vi "Func-엑셀 데이터를 그래프로 출력.vi"() -> ()   [LabVIEW 2015] (continued)
65\t64.9\t75.27\n65\t64.91\t75.268\n65\t64.92\t75.265\n65\t64.93\t75.262\n65\t64.94\t75.262\n65\t64.95\t75.256\n65\t64.96\t75.249\n65\t64.97\t75.245\n65\t64.98\t75.237\n65\t65\t75.229\n65\t64.96\t75.224\n65\t64.96\t75.22\n65\t64.96\t75.216\n65\t64.96\t75.208\n65\t64.96\t75.205\n65\t64.96\t75.201\n65\t64.96\t75.197\n65\t64.96\t75.188\n65\t64.96\t75.185\n65\t64.96\t75.182\n65\t64.96\t75.17\n65\t64.97\t75.163\n65\t64.97\t75.157\n65\t64.97\t75.149\n65\t64.97\t75.143\n65\t64.97\t75.135\n65\t64.97\t75.135\n65\t64.97\t75.134\n65\t64.97\t75.125\n65\t64.97\t75.123\n65\t64.97\t75.118\n65\t64.97\t75.114\n65\t64.97\t75.107\n65\t64.97\t75.099\n65\t64.97\t75.093\n65\t64.97\t75.088\n65\t64.97\t75.082\n65\t64.97\t75.077\n65\t64.97\t75.071\n65\t64.97\t75.065\n65\t64.97\t75.059\n65\t64.97\t75.055\n65\t64.97\t75.052\n65\t64.97\t75.045\n65\t64.97\t75.038\n65\t64.97\t75.037\n65\t64.97\t75.034\n65\t64.97\t75.028\n65\t64.97\t75.023\n65\t64.97\t75.021\n65\t64.97\t75.017\n65\t64.98\t75.007\n65\t64.98\t75\n65\t64.98\t74.998\n65\t64.98\t74.991\n65\t64.98\t74.981\n65\t64.98\t74.977\n65\t64.98\t74.97\n65\t64.98\t74.965\n65\t64.98\t74.957\n65\t64.98\t74.952\n65\t64.98\t74.95\n65\t64.98\t74.948\n65\t64.98\t74.945\n65\t64.98\t74.943\n65\t64.98\t74.938\n65\t64.98\t74.928\n65\t64.98\t74.923\n65\t64.98\t74.909\n65\t64.98\t74.903\n65\t64.98\t74.896\n65\t64.98\t74.894\n65\t64.98\t74.891\n65\t64.98\t74.884\n65\t64.98\t74.88\n65\t64.98\t74.881\n65\t64.98\t74.88\n65\t64.98\t74.871\n65\t64.98\t74.869\n65\t64.98\t74.87\n65\t64.98\t74.864\n65\t64.98\t74.858\n65\t65\t74.853\n65\t65\t74.849\n65\t65\t74.846\n65\t65\t74.836\n65\t65\t74.829\n65\t65\t74.824\n65\t65\t74.812\n65\t65\t74.809\n65\t65\t74.802\n65\t65\t74.798\n65\t65\t74.795\n65\t65\t74.789\n65\t65\t74.786\n65\t65\t74.782\n65\t65\t74.778\n65\t65\t74.771\n65\t65\t74.766\n65\t65\t74.764\n65\t65\t74.755\n65\t65\t74.748\n65\t65\t74.743\n65\t65\t74.742\n65\t65\t74.74\n65\t65\t74.736\n65\t65\t74.735\n65\t65\t74.732\n65\t65\t74.725\n65\t65\t74.717\n65\t65\t74.713\n65\t65\t74.707\n65\t65\t74.7\n65\t65\t74.693\n65\t65\t74.689\n65\t65\t74.688\n65\t65\t74.684\n65\t65\t74.675\n65\t65\t74.672\n65\t65\t74.671\n65\t65\t74.666\n65\t65\t74.662\n65\t65\t74.657\n65\t65\t74.654\n65\t65\t74.652\n65\t65\t74.647\n65\t65\t74.638\n65\t65\t74.634\n65\t65\t74.628\n65\t65\t74.622\n65\t65\t74.616\n65\t65\t74.612\n65\t65\t74.602\n65\t65\t74.598\n65\t65\t74.596\n65\t65\t74.587\n65\t65\t74.581\n65\t65\t74.573\n65\t65\t74.572\n65\t65\t74.568\n65\t65\t74.561\n65\t65\t74.562\n65\t65\t74.56\n65\t65\t74.559\n65\t65\t74.559\n65\t65\t74.551\n65\t65\t74.547\n65\t65\t74.538\n65\t65\t74.537\n65\t65\t74.53\n65\t65\t74.523\n65\t65\t74.52\n65\t65\t74.513\n65\t65\t74.512\n65\t65\t74.506\n65\t65\t74.504\n65\t65\t74.5\n65\t65\t74.494\n65\t65\t74.489\n65\t65\t74.484\n65\t65\t74.477\n65\t65\t74.471\n65\t65\t74.467\n65\t65\t74.466\n65\t65\t74.462\n65\t65\t74.461\n65\t65\t74.454\n65\t65\t74.447\n65\t65\t74.444\n65\t65\t74.436\n65\t65\t74.431\n65\t65\t74.422\n65\t65\t74.42\n65\t65\t74.413\n65\t65\t74.41\n65\t65\t74.405\n65\t65\t74.403\n65\t65\t74.401\n65\t65\t74.395\n65\t65\t74.392\n65\t65\t74.386\n65\t65\t74.382\n65\t65\t74.377\n65\t65\t74.373\n65\t65\t74.368\n65\t65\t74.366\n65\t65\t74.362\n65\t65\t74.356\n65\t65\t74.355\n65\t65\t74.35\n65\t65\t74.347\n65\t65\t74.341\n65\t65\t74.336\n65\t65\t74.332\n65\t65\t74.328\n65\t65\t74.323\n65\t65\t74.323\n65\t65\t74.322\n65\t65\t74.315\n65\t65\t74.311\n65\t65\t74.301\n65\t65\t74.298\n65\t65\t74.292\n65\t65\t74.29\n65\t65\t74.289\n65\t65\t74.285\n65\t65\t74.279\n65\t65\t74.276\n65\t65\t74.27\n65\t65\t74.264\n65\t65\t74.257\n65\t65\t74.251\n65\t65\t74.247\n65\t65\t74.242\n65\t65\t74.238\n65\t65\t74.229\n65\t65\t74.23\n65\t65\t74.228\n65\t65\t74.229\n65\t65\t74.226\n65\t65\t74.222\n65\t65\t74.219\n65\t65\t74.212\n65\t65\t74.211\n65\t65\t74.201\n65\t65\t74.198\n65\t65\t74.196\n65\t65\t74.19\n65\t65\t74.186\n65\t65\t74.183\n65\t65\t74.179\n65\t65\t74.176\n65\t65\t74.17\n65\t65\t74.17\n65\t65\t74.165\n65\t65\t74.159\n65\t65\t74.155\n65\t65\t74.148\n65\t65\t74.139\n65\t65\t74.136\n65\t65\t74.134\n65\t65\t74.13\n65\t65\t74.127\n65\t65\t74.124\n65\t65\t74.123\n65\t65\t74.122\n65\t65\t74.116\n65\t65\t74.112\n65\t65\t74.108\n65\t65\t74.101\n65\t65\t74.099\n65\t65\t74.092\n65\t65\t74.088\n65\t65\t74.083\n65\t65\t74.078\n65\t65\t74.075\n65\t65\t74.074\n65\t65\t74.073\n65\t65\t74.068\n65\t65\t74.066\n65\t65\t74.061\n65\t65\t74.061\n65\t65\t74.053\n65\t65\t74.049\n65\t65\t74.049\n65\t65\t74.047\n65\t65\t74.045\n65\t65\t74.038\n65\t65\t74.037\n65\t65\t74.033\n65\t65\t74.025\n65\t65\t74.021\n65\t65\t74.016\n65\t65\t74.015\n65\t65\t74.011\n65\t65\t74.003\n65\t65\t74\n65\t65\t73.996\n65\t65\t73.987\n65\t65\t73.983\n65\t65\t73.982\n65\t65\t73.977\n65\t65\t73.975\n65\t65\t73.968\n65\t65\t73.963\n65\t65\t73.96\n65\t65\t73.956\n65\t65\t73.952\n65\t65\t73.949\n65\t65\t73.946\n65\t65\t73.946\n65\t65\t73.94\n65\t65\t73.933\n65\t65\t73.933\n65\t65\t73.928\n65\t65\t73.923\n65\t65\t73.923\n65\t65\t73.919\n65\t65\t73.916\n65\t65\t73.908\n65\t65\t73.904\n65\t65\t73.902\n65\t65\t73.895\n65\t65\t73.895\n65\t65\t73.892\n65\t65\t73.89\n65\t65\t73.889\n65\t65\t73.886\n65\t65\t73.884\n65\t65\t73.879\n65\t65\t73.873\n65\t65\t73.87\n65\t65\t73.864\n65\t65\t73.858\n65\t65\t73.855\n65\t65\t73.848\n65\t65\t73.845\n65\t65\t73.841\n65\t65\t73.839\n65\t65\t73.835\n65\t65\t73.833\n65\t65\t73.83\n65\t65\t73.831\n65\t65\t73.827\n65\t65\t73.823\n65\t65\t73.82\n65\t65\t73.809\n65\t65\t73.804\n65\t65\t73.798\n65\t65\t73.793\n65\t65\t73.787\n65\t65\t73.787\n65\t65\t73.788\n65\t65\t73.787\n65\t65\t73.784\n65\t65\t73.781\n65\t65\t73.78\n65\t65\t73.773\n65\t65\t73.766\n65\t65\t73.761\n65\t65\t73.757\n65\t65\t73.752\n65\t65\t73.747\n65\t65\t73.744\n65\t65\t73.743\n65\t65\t73.739\n65\t65\t73.736\n65\t65\t73.734\n65\t65\t73.73\n65\t65\t73.73\n65\t65\t73.729\n65\t65\t73.727\n65\t65\t73.724\n65\t65\t73.721\n65\t65\t73.716\n65\t65\t73.71\n65\t65\t73.705\n65\t65\t73.701\n65\t65\t73.697\n65\t65\t73.697\n65\t65\t73.697\n65\t65\t73.691\n65\t65\t73.686\n65\t65\t73.68\n65\t65\t73.675\n65\t65\t73.669\n65\t65\t73.664\n65\t65\t73.663\n65\t65\t73.662\n65\t65\t73.658\n65\t65\t73.654\n65\t65\t73.655\n65\t65\t73.649\n65\t65\t73.648\n65\t65\t73.644\n65\t65\t73.642\n65\t65\t73.641\n65\t65\t73.634\n65\t65\t73.632\n65\t65\t73.629\n65\t65\t73.625\n65\t65\t73.621\n65\t65\t73.614\n65\t65\t73.614\n65\t65\t73.61\n65\t65\t73.606\n65\t65\t73.605\n65\t65\t73.602\n65\t65\t73.6\n65\t65\t73.592\n65\t65\t73.585\n65\t65\t73.581\n65\t65\t73.572\n65\t65\t73.571\n65\t65\t73.572\n65\t65\t73.569\n65\t65\t73.572\n65\t65\t73.575\n65\t65\t73.576\n65\t65\t73.573\n65\t65\t73.572\n65\t65\t73.57\n65\t65\t73.562\n65\t65\t73.555\n65\t65\t73.549\n65\t65\t73.544\n65\t65\t73.539\n65\t65\t73.535\n65\t65\t73.537\n65\t65\t73.53\n65\t65\t73.528\n65\t65\t73.524\n65\t65\t73.518\n65\t65\t73.513\n65\t65\t73.51\n65\t65\t73.509\n65\t65\t73.506\n65\t65\t73.501\n65\t65\t73.497\n65\t65\t73.493\n65\t65\t73.486\n65\t65\t73.482\n65\t65\t73.477\n65\t65\t73.479\n65\t65\t73.474\n65\t65\t73.475\n65\t65\t73.474\n65\t65\t73.471\n65\t65\t73.471\n65\t65\t73.466\n65\t65\t73.46\n65\t65\t73.457\n65\t65\t73.45\n65\t65\t73.444\n65\t65\t73.442\n65\t65\t73.443\n65\t65\t73.446\n65\t65\t73.445\n65\t65\t73.443\n65\t65\t73.439\n65\t65\t73.434\n65\t65\t73.427\n65\t65\t73.421\n65\t65\t73.413\n65\t65\t73.407\n65\t65\t73.41\n65\t65\t73.405\n65\t65\t73.406\n65\t65\t73.406\n65\t65\t73.408\n65\t65\t73.407\n65\t65\t73.403\n65\t65\t73.402\n65\t65\t73.396\n65\t65\t73.393\n65\t65\t73.389\n65\t65\t73.386\n65\t65\t73.382\n65\t65\t73.377\n65\t65\t73.373\n65\t65\t73.37\n65\t65\t73.365\n65\t65\t73.364\n65\t65\t73.363\n65\t65\t73.361\n65\t65\t73.359\n65\t65\t73.356\n65\t65\t73.355\n65\t65\t73.354\n65\t65\t73.351\n65\t65\t73.345\n65\t65\t73.343\n65\t65\t73.338\n65\t65\t73.326\n65\t65\t73.32\n65\t65\t73.314\n65\t65\t73.315\n65\t65\t73.312\n65\t65\t73.313\n65\t65\t73.316\n65\t65\t73.31\n65\t65\t73.305\n65\t65\t73.299\n65\t65\t73.294\n65\t65\t73.286\n65\t65\t73.282\n65\t65\t73.284\n65\t65\t73.283\n65\t65\t73.282\n65\t65\t73.284\n65\t65\t73.28\n65\t65\t73.279\n65\t65\t73.277\n65\t65\t73.275\n65\t65\t73.273\n65\t65\t73.266\n65\t65\t73.265\n65\t65\t73.263\n65\t65\t73.257\n65\t65\t73.251\n65\t65\t73.246\n65\t65\t73.244\n65\t65\t73.242\n65\t65\t73.238\n65\t65\t73.236\n65\t65\t73.236\n65\t65\t73.233\n65\t65\t73.232\n65\t65\t73.227\n65\t65\t73.226\n65\t65\t73.219\n65\t65\t73.213\n65\t65\t73.209\n65\t65\t73.205\n65\t65\t73.204\n65\t65\t73.201\n65\t65\t73.201\n65\t65\t73.205\n65\t65\t73.2\n65\t65\t73.195\n65\t65\t73.194\n65\t65\t73.19\n65\t65\t73.187\n65\t65\t73.181\n65\t65\t73.182\n65\t65\t73.183\n65\t65\t73.18\n65\t65\t73.175\n65\t65\t73.173\n65\t65\t73.17\n65\t65\t73.168\n65\t65\t73.164\n65\t65\t73.165\n65\t65\t73.162\n65\t65\t73.158\n65\t65\t73.156\n65\t65\t73.155\n65\t65\t73.154\n65\t65\t73.15\n65\t65\t73.148\n65\t65\t73.148\n65\t65\t73.142\n65\t65\t73.139\n65\t65\t73.136\n65\t65\t73.127\n65\t65\t73.124\n65\t65\t73.122\n65\t65\t73.121\n65\t65\t73.113\n65\t65\t73.109\n65\t65\t73.109\n65\t65\t73.108\n65\t65\t73.101\n65\t65\t73.101\n65\t65\t73.1\n65\t65\t73.098\n65\t65\t73.101\n65\t65\t73.097\n65\t65\t73.098\n65\t65\t73.097\n65\t65\t73.098\n65\t65\t73.094\n65\t65\t73.089\n65\t65\t73.086\n65\t65\t73.078\n65\t65\t73.071\n65\t65\t73.068\n65\t65\t73.062\n65\t65\t73.056\n65\t65\t73.055\n65\t65\t73.052\n65\t65\t73.05\n65\t65\t73.047\n65\t65\t73.048\n65\t65\t73.048\n65\t65\t73.043\n65\t65\t73.037\n65\t65\t73.033\n65\t65\t73.028\n65\t65\t73.023\n65\t65\t73.02\n65\t65\t73.018\n65\t65\t73.02\n65\t65\t73.021\n65\t65\t73.017\n65\t65\t73.013\n65\t65\t73.015\n65\t65\t73.011\n65\t65\t73.009\n65\t65\t73\n65\t65\t72.997\n65\t65\t72.996\n65\t65\t72.988\n65\t65\t72.988\n65\t65\t72.986\n65\t65\t72.988\n65\t65\t72.988\n65\t65\t72.984\n65\t65\t72.983\n65\t65\t72.979\n65\t65\t72.977\n65\t65\t72.978\n65\t65\t72.976\n65\t65\t72.975\n65\t65\t72.972\n65\t65\t72.971\n65\t65\t72.968\n65\t65\t72.963\n65\t65\t72.96\n65\t65\t72.96\n65\t65\t72.957\n65\t65\t72.955\n65\t65\t72.949\n65\t65\t72.948\n65\t65\t72.945\n65\t65\t72.94\n65\t65\t72.936\n65\t65\t72.935\n65\t65\t72.935\n65\t65\t72.934\n65\t65\t72.932\n65\t65\t72.929\n65\t65\t72.932\n65\t65\t72.93\n65\t65\t72.928\n65\t65\t72.922\n65\t65\t72.917\n65\t65\t72.913\n65\t65\t72.909\n65\t65\t72.905\n65\t65\t72.902\n65\t65\t72.901\n65\t65\t72.901\n65\t65\t72.9\n65\t65\t72.893\n65\t65\t72.894\n65\t65\t72.891\n65\t65\t72.896\n65\t65\t72.893\n65\t65\t72.891\n65\t65\t72.891\n65\t65\t72.881\n65\t65\t72.881\n65\t65\t72.871\n65\t65\t72.871\n65\t65\t72.87\n65\t65\t72.87\n65\t65\t72.872\n65\t65\t72.868\n65\t65\t72.866\n65\t65\t72.863\n65\t65\t72.858\n65\t65\t72.854\n65\t65\t72.845\n65\t65\t72.845\n65\t65\t72.84\n65\t65\t72.838\n65\t65\t72.834\n65\t65\t72.833\n65\t65\t72.833\n65\t65\t72.829\n65\t65\t72.828\n65\t65\t72.822\n65\t65\t72.825\n65\t65\t72.824\n65\t65\t72.818\n65\t65\t72.816\n65\t65\t72.817\n65\t65\t72.819\n65\t65\t72.814\n65\t65\t72.809\n65\t65\t72.81\n65\t65\t72.811\n65\t65\t72.805\n65\t65\t72.796\n65\t65\t72.798\n65\t65\t72.796\n65\t65\t72.793\n65\t65\t72.786\n65\t65\t72.78\n65\t65\t72.777\n65\t65\t72.772\n65\t65\t72.772\n65\t65\t72.771\n65\t65\t72.773\n65\t65\t72.771\n65\t65\t72.776\n65\t65\t72.772\n65\t65\t72.768\n65\t65\t72.767\n65\t65\t72.761\n65\t65\t72.759\n65\t65\t72.755\n65\t65\t72.753\n65\t65\t72.751\n65\t65\t72.748\n65\t65\t72.751\n65\t65\t72.753\n65\t65\t72.751\n65\t65\t72.749\n65\t65\t72.745\n65\t65\t72.738\n65\t65\t72.733\n65\t65\t72.73\n65\t65\t72.724\n65\t65\t72.721\n65\t65\t72.721\n65\t65\t72.721\n65\t65\t72.719\n65\t65\t72.716\n65\t65\t72.72\n65\t65\t72.722\n65\t65\t72.72\n65\t65\t72.716\n65\t65\t72.717\n65\t65\t72.716\n65\t65\t72.709\n65\t65\t72.705\n65\t65\t72.705\n65\t65\t72.703\n65\t65\t72.697\n65\t65\t72.692\n65\t65\t72.691\n65\t65\t72.687\n65\t65\t72.682\n65\t65\t72.684\n65\t65\t72.689\n65\t65\t72.689\n65\t65\t72.682\n65\t65\t72.681\n65\t65\t72.68\n65\t65\t72.679\n65\t65\t72.673\n65\t65\t72.67\n65\t65\t72.671\n65\t65\t72.671\n65\t65\t72.667\n65\t65\t72.662\n65\t65\t72.657\n65\t65\t72.653\n65\t65\t72.652\n65\t65\t72.648\n65\t65\t72.647\n65\t65\t72.641\n65\t65\t72.644\n65\t65\t72.641\n65\t65\t72.64\n65\t65\t72.642\n65\t65\t72.639\n65\t65\t72.638\n65\t65\t72.636\n65\t65\t72.635\n65\t65\t72.632\n65\t65\t72.625\n65\t65\t72.62\n65\t65\t72.623\n65\t65\t72.62\n65\t65\t72.62\n65\t65\t72.619\n65\t65\t72.618\n65\t65\t72.616\n65\t65\t72.613\n65\t65\t72.61\n65\t65\t72.607\n65\t65\t72.605\n65\t65\t72.602\n65\t65\t72.601\n65\t65\t72.597\n65\t65\t72.595\n65\t65\t72.593\n65\t65\t72.59\n65\t65\t72.588\n65\t65\t72.585\n65\t65\t72.586\n65\t65\t72.584\n65\t65\t72.582\n65\t65\t72.581\n65\t65\t72.582\n65\t65\t72.581\n65\t65\t72.575\n65\t65\t72.572\n65\t65\t72.574\n65\t65\t72.57\n65\t65\t72.565\n65\t65\t72.566\n65\t65\t72.565\n65\t65\t72.562\n65\t65\t72.56\n65\t65\t72.555\n65\t65\t72.555\n65\t65\t72.551\n65\t65\t72.548\n65\t65\t72.549\n65\t65\t72.543\n65\t65\t72.544\n65\t65\t72.539\n65\t65\t72.54\n65\t65\t72.539\n65\t65\t72.536\n65\t65\t72.532\n65\t65\t72.529\n65\t65\t72.532\n65\t65\t72.526\n65\t65\t72.524\n65\t65\t72.522\n65\t65\t72.517\n65\t65\t72.519\n65\t65\t72.512\n65\t65\t72.514\n65\t65\t72.51\n65\t65\t72.51\n65\t65\t72.512\n65\t65\t72.506\n65\t65\t72.506\n65\t65\t72.501\n65\t65\t72.5\n65\t65\t72.493\n65\t65\t72.493\n65\t65\t72.493\n65\t65\t72.491\n65\t65\t72.493\n65\t65\t72.491\n65\t65\t72.492\n65\t65\t72.492\n65\t65\t72.488\n65\t65\t72.485\n65\t65\t72.478\n65\t65\t72.475\n65\t65\t72.47\n65\t65\t72.465\n65\t65\t72.467\n65\t65\t72.466\n65\t65\t72.467\n65\t65\t72.467\n65\t65\t72.466\n65\t65\t72.468\n65\t65\t72.464\n65\t65\t72.463\n65\t65\t72.463\n65\t65\t72.459\n65\t65\t72.452\n65\t65\t72.448\n65\t65\t72.445\n65\t65\t72.443\n65\t65\t72.44\n65\t65\t72.437\n65\t65\t72.439\n65\t65\t72.437\n65\t65\t72.434\n65\t65\t72.43\n65\t65\t72.428\n65\t65\t72.431\n65\t65\t72.434\n65\t65\t72.431\n65\t65\t72.429\n65\t65\t72.429\n65\t65\t72.424\n65\t65\t72.422\n65\t65\t72.421\n65\t65\t72.421\n65\t65\t72.42\n65\t65\t72.416\n65\t65\t72.418\n65\t65\t72.414\n65\t65\t72.408\n65\t65\t72.405\n65\t65\t72.406\n65\t65\t72.405\n65\t65\t72.399\n65\t65\t72.398\n65\t65\t72.4\n65\t65\t72.401\n65\t65\t72.397\n65\t65\t72.398\n65\t65\t72.402\n65\t65\t72.402\n65\t65\t72.396\n65\t65\t72.391\n65\t65\t72.391\n65\t65\t72.385\n65\t65\t72.379\n65\t65\t72.373\n65\t65\t72.37\n65\t65\t72.368\n65\t65\t72.367\n65\t65\t72.365\n65\t65\t72.366\n65\t65\t72.366\n65\t65\t72.367\n65\t65\t72.366\n65\t65\t72.364\n65\t65\t72.363\n65\t65\t72.36\n65\t65\t72.359\n65\t65\t72.358\n65\t65\t72.356\n65\t65\t72.355\n65\t65\t72.356\n65\t65\t72.358\n65\t65\t72.355\n65\t65\t72.352\n65\t65\t72.353\n65\t65\t72.345\n65\t65\t72.342\n65\t65\t72.336\n65\t65\t72.338\n65\t65\t72.337\n65\t65\t72.332\n65\t65\t72.331\n65\t65\t72.325\n65\t65\t72.324\n65\t65\t72.317\n65\t65\t72.316\n65\t65\t72.314\n65\t65\t72.318\n65\t65\t72.319\n65\t65\t72.317\n65\t65\t72.317\n65\t65\t72.312\n65\t65\t72.307\n65\t65\t72.303\n65\t65\t72.302\n65\t65\t72.299\n65\t65\t72.298\n65\t65\t72.295\n65\t65\t72.294\n65\t65\t72.296\n65\t65\t72.299\n65\t65\t72.3\n65\t65\t72.3\n65\t65\t72.298\n65\t65\t72.295\n65\t65\t72.293\n65\t65\t72.288\n65\t65\t72.281\n65\t65\t72.275\n65\t65\t72.28\n65\t65\t72.279\n65\t65\t72.276\n65\t65\t72.273\n65\t65\t72.271\n65\t65\t72.27\n65\t65\t72.268\n65\t65\t72.266\n65\t65\t72.264\n65\t65\t72.265\n65\t65\t72.271\n65\t65\t72.271\n65\t65\t72.266\n65\t65\t72.267\n65\t65\t72.267\n65\t65\t72.266\n65\t65\t72.257\n65\t65\t72.253\n65\t65\t72.254\n65\t65\t72.253\n65\t65\t72.248\n65\t65\t72.245\n65\t65\t72.245\n65\t65\t72.247\n65\t65\t72.243\n65\t65\t72.241\n65\t65\t72.239\n65\t65\t72.239\n65\t65\t72.24\n65\t65\t72.236\n65\t65\t72.239\n65\t65\t72.237\n65\t65\t72.239\n65\t65\t72.238\n65\t65\t72.236\n65\t65\t72.236\n65\t65\t72.229\n65\t65\t72.231\n65\t65\t72.231\n65\t65\t72.225\n65\t65\t72.22\n65\t65\t72.218\n65\t65\t72.217\n65\t65\t72.21\n65\t65\t72.205\n65\t65\t72.203\n65\t65\t72.204\n65\t65\t72.204\n65\t65\t72.204\n65\t65\t72.206\n65\t65\t72.205\n65\t65\t72.207\n65\t65\t72.209\n65\t65\t72.206\n65\t65\t72.204\n65\t65\t72.202\n65\t65\t72.2\n65\t65\t72.197\n65\t65\t72.19\n65\t65\t72.188\n65\t65\t72.189\n65\t65\t72.186\n65\t65\t72.18\n65\t65\t72.18\n65\t65\t72.178\n65\t65\t72.176\n65\t65\t72.173\n65\t65\t72.172\n65\t65\t72.175\n65\t65\t72.172\n65\t65\t72.172\n65\t65\t72.169\n65\t65\t72.17\n65\t65\t72.169\n65\t65\t72.166\n65\t65\t72.164\n65\t65\t72.16\n65\t65\t72.163\n65\t65\t72.161\n65\t65\t72.159\n65\t65\t72.162\n65\t65\t72.158\n65\t65\t72.162\n65\t65\t72.158\n65\t65\t72.152\n65\t65\t72.149\n65\t65\t72.142\n65\t65\t72.143\n65\t65\t72.14\n65\t65\t72.137\n65\t65\t72.137\n65\t65\t72.137\n65\t65\t72.138\n65\t65\t72.136\n65\t65\t72.134\n65\t65\t72.134\n65\t65\t72.135\n65\t65\t72.135\n65\t65\t72.13\n65\t65\t72.129\n65\t65\t72.128\n65\t65\t72.123\n65\t65\t72.119\n65\t65\t72.117\n65\t65\t72.116\n65\t65\t72.113\n65\t65\t72.108\n65\t65\t72.109\n65\t65\t72.107\n65\t65\t72.105\n65\t65\t72.105\n65\t65\t72.102\n65\t65\t72.104\n65\t65\t72.102\n65\t65\t72.101\n65\t65\t72.1\n65\t65\t72.099\n65\t65\t72.1\n65\t65\t72.096\n65\t65\t72.095\n65\t65\t72.095\n65\t65\t72.088\n65\t65\t72.089\n65\t65\t72.089\n65\t65\t72.091\n65\t65\t72.089\n65\t65\t72.087\n65\t65\t72.086\n65\t65\t72.086\n65\t65\t72.084\n65\t65\t72.083\n65\t65\t72.084\n65\t65\t72.084\n65\t65\t72.087\n65\t65\t72.083\n65\t65\t72.083\n65\t65\t72.078\n65\t65\t72.073\n65\t65\t72.069\n65\t65\t72.065\n65\t65\t72.064\n65\t65\t72.063\n65\t65\t72.061\n65\t65\t72.06\n65\t65\t72.06\n65\t65\t72.057\n65\t65\t72.056\n65\t65\t72.051\n65\t65\t72.052\n65\t65\t72.051\n65\t65\t72.048\n65\t65\t72.049\n65\t65\t72.049\n65\t65\t72.046\n65\t65\t72.042\n65\t65\t72.045\n65\t65\t72.045\n65\t65\t72.043\n65\t65\t72.043\n65\t65\t72.044\n65\t65\t72.041\n65\t65\t72.039\n65\t65\t72.034\n65\t65\t72.036\n65\t65\t72.03\n65\t65\t72.027\n65\t65\t72.03\n65\t65\t72.026\n65\t65\t72.027\n65\t65\t72.021\n65\t65\t72.02\n65\t65\t72.016\n65\t65\t72.015\n65\t65\t72.014\n65\t65\t72.016\n65\t65\t72.016\n65\t65\t72.016\n65\t65\t72.017\n65\t65\t72.011\n65\t65\t72.012\n65\t65\t72.008\n65\t65\t72.006\n65\t65\t72.004\n65\t65\t72.005\n65\t65\t72.004\n65\t65\t72.004\n65\t65\t72.001\n65\t65\t71.998\n65\t65\t72\n65\t65\t71.996\n65\t65\t71.996\n65\t65\t71.992\n65\t65\t71.991\n65\t65\t71.994\n65\t65\t71.989\n65\t65\t71.984\n65\t65\t71.986\n65\t65\t71.984\n65\t65\t71.984\n65\t65\t71.983\n65\t65\t71.985\n65\t65\t71.988\n65\t65\t71.981\n65\t65\t71.977\n65\t65\t71.976\n65\t65\t71.976\n65\t65\t71.972\n65\t65\t71.971\n65\t65\t71.974\n65\t65\t71.977\n65\t65\t71.975\n65\t65\t71.972\n65\t65\t71.967\n65\t65\t71.963\n65\t65\t71.961\n65\t65\t71.957\n65\t65\t71.957\n65\t65\t71.956\n65\t65\t71.964\n65\t65\t71.963\n65\t65\t71.963\n65\t65\t71.961\n65\t65\t71.954\n65\t65\t71.951\n65\t65\t71.943\n65\t65\t71.942\n65\t65\t71.942\n65\t65\t71.938\n65\t65\t71.944\n65\t65\t71.947\n65\t65\t71.947\n65\t65\t71.948\n65\t65\t71.946\n65\t65\t71.946\n65\t65\t71.943\n65\t65\t71.94\n65\t65\t71.938\n65\t65\t71.935\n65\t65\t71.93\n65\t65\t71.93\n65\t65\t71.927\n65\t65\t71.926\n65\t65\t71.925\n65\t65\t71.925\n65\t65\t71.927\n65\t65\t71.927\n65\t65\t71.925\n65\t65\t71.926\n65\t65\t71.921\n65\t65\t71.919\n65\t65\t71.917\n65\t65\t71.914\n65\t65\t71.916\n65\t65\t71.912\n65\t65\t71.915\n65\t65\t71.911\n65\t65\t71.911\n65\t65\t71.907\n65\t65\t71.903\n65\t65\t71.902\n65\t65\t71.899\n65\t65\t71.9\n65\t65\t71.902\n65\t65\t71.904\n65\t65\t71.904\n65\t65\t71.901\n65\t65\t71.902\n65\t65\t71.899\n65\t65\t71.895\n65\t65\t71.894\n65\t65\t71.893\n65\t65\t71.894\n65\t65\t71.889\n65\t65\t71.888\n65\t65\t71.888\n65\t65\t71.887\n65\t65\t71.891\n65\t65\t71.892\n65\t65\t71.891\n65\t65\t71.892\n65\t65\t71.887\n65\t65\t71.885\n65\t65\t71.88\n65\t65\t71.877\n65\t65\t71.878\n65\t65\t71.875\n65\t65\t71.877\n65\t65\t71.875\n65\t65\t71.873\n65\t65\t71.873\n65\t65\t71.87\n65\t65\t71.868\n65\t65\t71.866\n65\t65\t71.864\n65\t65\t71.862\n65\t65\t71.861\n65\t65\t71.858\n65\t65\t71.857\n65\t65\t71.856\n65\t65\t71.861\n65\t65\t71.858\n65\t65\t71.857\n65\t65\t71.855\n65\t65\t71.855\n65\t65\t71.85\n65\t65\t71.847\n65\t65\t71.847\n65\t65\t71.841\n
